vi "Get Data.vi"(8 "Error in":errorcluster) -> (0 "Error out":errorcluster, 2 "Message FPGA":T1)   [LabVIEW 2021]
uses:
  Typedefs/Message FPGA.ctl
  Typedefs/Q Action.ctl
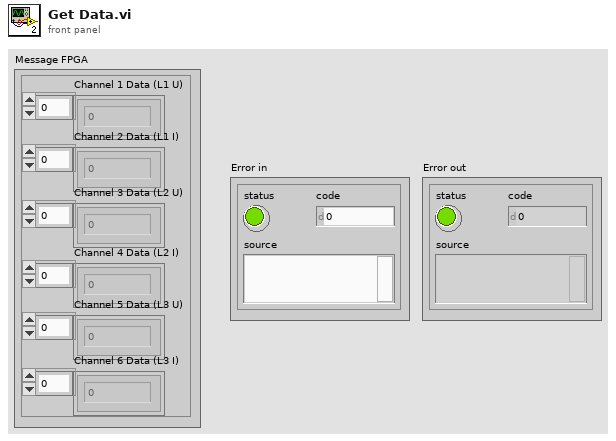
[diagram p1: front panel]
types:
  T1 = typedef "Message FPGA.ctl" = cluster{"Channel 1 Data (L1 U)":dbl[], "Channel 2 Data (L1 I)":dbl[], "Channel 3 Data (L2 U)":dbl[], "Channel 4 Data (L2 I)":dbl[], "Channel 5 Data (L3 U)":dbl[], "Channel 6 Data (L3 I)":dbl[]}
  T2 = typedef "Q Action.ctl" = enum16{"Obtain Queue", "Enqueue", "Dequeue", "Close"}
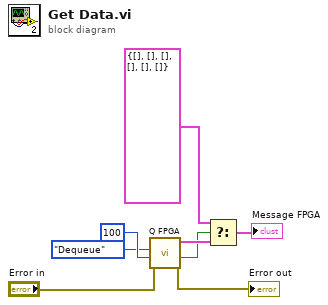
[diagram p0: block diagram]
diagram:
  n1 = call "Q FPGA.vi"("Error in"="Error in", "Timeout"=100, "Action"=Q_Action."Dequeue") -> ("Error out"=→"Error out":errorcluster, "Timed out?"=w6:bool, "Message FPGA out"=w7:T1)  [unwired: 6 in]
  n2 = Select(t=T1 {"Channel 1 Data (L1 U)"=[], "Channel 2 Data (L1 I)"=[], "Channel 3 Data (L2 U)"=[], "Channel 4 Data (L2 I)"=[], "Channel 5 Data (L3 U)"=[], "Channel 6 Data (L3 I)"=[]}, s=w6, f=w7) -> (s? t:f=→"Message FPGA":T1)
